vi "Global_HW_Data Out.vi"() -> ()   [LabVIEW 2017, in "Sonar.lvlib"]
uses:
  Sonar.lvlib
panel:
  in  "HW_Sonar Distance":dbl
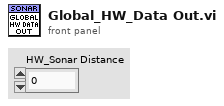
[diagram p1: front panel]
diagram:
